vi "Set_Prop_Write_Create_Const.vi"(8 "error in (no error)":errorcluster, 10 "Value":variant, 11 "PropertyItem in":refnum<vi>) -> (0 "error out":errorcluster)   [LabVIEW 2025]
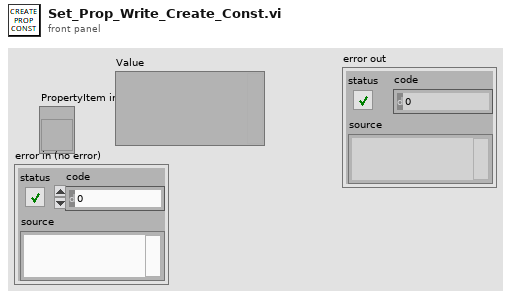
[diagram p1: front panel]
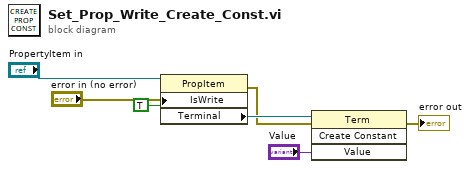
[diagram p0: block diagram]
diagram:
  n1 = property class="PropItem"(reference="PropertyItem in", error in="error in (no error)", "IsWrite"=TRUE ("Is Write")) -> (error out=w3:errorcluster, "Terminal"=w6:refnum<vi>)  [unwired: 1 out]
  n2 = invoke class="Term" method="Create Constant"(reference=w6, error in=w3, "Value"="Value") -> (error out=→"error out":errorcluster)  [unwired: 1 in, 3 out]
